vi "write_params.vi"(8 "error in (no error)":errorcluster, 10 "params":T1={"alphas"=[0.1, 1.0, 10.0], "fit_intercept"=TRUE, "normalize"=FALSE, "scoring"="None", "cv"=5.0, "gcv_mode"="auto", "store_cv_values"=FALSE, "alpha_per_target"=FALSE}, 11 "RidgeCV in":refnum<class "RidgeCV.lvclass">) -> (0 "error out":errorcluster, 3 "RidgeCV out":refnum<class "RidgeCV.lvclass">)   [LabVIEW 2020, in "RidgeCV.lvclass"]
uses:
  RidgeCV.lvclass
  Controls/ridge_cv_params.ctl
  RidgeCV.lvclass/RidgeCV.ctl
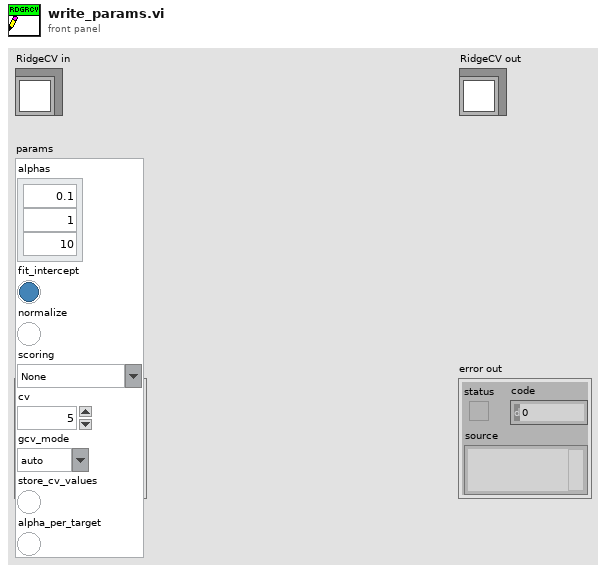
[diagram p1: front panel]
types:
  T1 = typedef "ridge_cv_params.ctl" = cluster{"alphas":dbl[], "fit_intercept":bool, "normalize":bool, "scoring":string, "cv":dbl, "gcv_mode":string, "store_cv_values":bool, "alpha_per_target":bool}
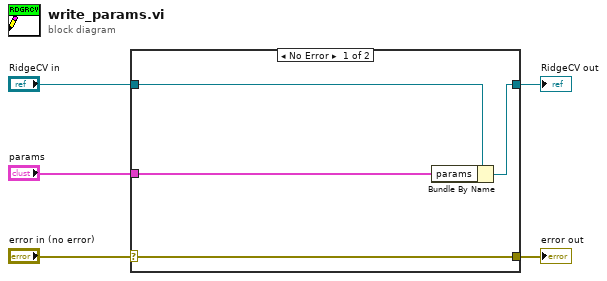
[diagram p0: block diagram]
diagram:
  n1 = case shown="No Error" "error in (no error)" {
    selector: "error in (no error)" -> [w9 w10]
    tunnel: [w9 w10] -> w4
    tunnel: [w7 w11] -> w2
    tunnel: "RidgeCV in" -> [w8 w11]
    tunnel: "params" -> [w6 _]
    frame No Error {
      n2 = Bundle By Name(cluster=w8, "params"=w6) -> (w7:refnum<class "RidgeCV.lvclass">)
    }
    frame Error {
    }
  }
  "error out" <- w4
  "RidgeCV out" <- w2
